vi "一体站流程自动启动.vi"(11 "参数":T1={"是否启用仪器"=FALSE, "CODMn"={"启动测量模式"={"测量模式"=enum."水样测量"}, "确定按钮"=TRUE}, "采水模式"=enum."使用采水泵"}) -> ()   [LabVIEW 2016, in "PLC.lvlib"]
uses:
  PLC.lvlib
panel:
  out "枚举":enum16{"初始化", "采配水启动", "等待", "配水", "排水", "结束"}(ring)
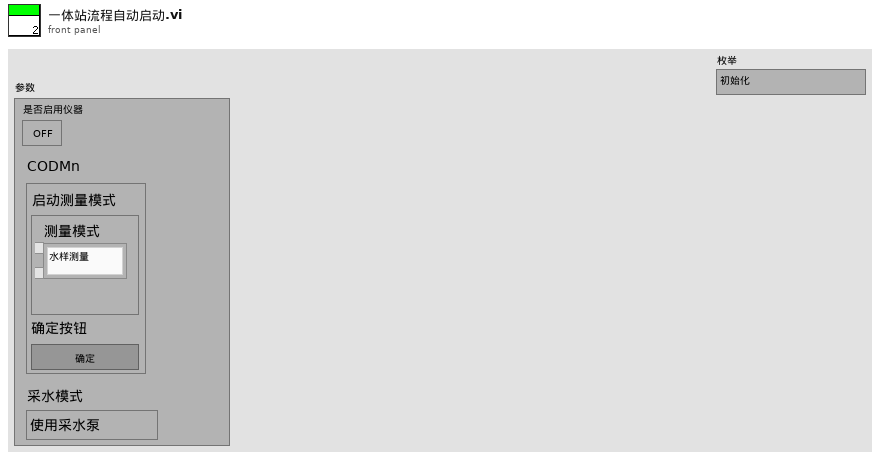
[diagram p1: front panel]
types:
  T1 = cluster{"是否启用仪器":bool, "CODMn":cluster{"启动测量模式":cluster{"测量模式":enum16{"水样测量", "标样核查", "零点核查", "加标回收", "平行样", "校零", "校标"}}, "确定按钮":bool}, "采水模式":enum16{"使用采水泵", "不使用采水泵"}}
  T2 = cluster{"命令":string, cluster{"starting address":u16, "holding register value":u16}}
  T3 = enum16{"待机", "启动氨氮", "氨氮测量中", "启动总磷", "总磷测量中", "结束"}
  T4 = cluster{"站号":u16, "量程切换":enum32{"H", "L", "AUTO"}, "控制命令":enum16{"启动测量", "标样核查", "零点核查", "跨度核查", "空白测试", "平行样测试", "加标回收", "空白校准", "标样校准", "初始化（清洗）", "停止测试", "仪器重启", "校时", "模式设置", "测量间隔设置", "盲样测试"}, "模式设置":enum16{"待机", "连续模式", "周期模式", "定点模式", "受控模式", "手动模式"}, "测量间隔":u16}
  T5 = cluster{"时间标识":timestamp, "设备":string, "日志信息":string}
  T6 = cluster{"测量模式":enum16{"待机", "水样测试", "标样核查", "零点核查", "跨度核查", "空白测试", "平行样测试", "加标回收", "空白校准", "标样校准", "初始化（清洗）"}, "数据标记表":string, "测量时间":dbl}
  T7 = enum16{"待机", "水样测试", "标样核查", "零点核查", "跨度核查", "空白测试", "平行样测试", "加标回收", "空白校准", "标样校准", "初始化（清洗）"}
  T8 = cluster{"R0":i16, "R1":i16, "R2":i16, "R3":i16, "R4":i16, "R5":i16, "R6":i16, "R7":i16, "R8":i16, "R9":i16, "R10":i16, "R11":i16, "R12":i16, "R13":i16, "R14":i16, "R15":i16, "R16":i16, "R17":i16, "R18":i16, "R19":i16, "R20":i16, "R21":i16, "R22":i16}
  T9 = enum32{"Bad", "Idle", "Run top level", "Running"}
  T10 = cluster{"测量模式":enum16{"水样测量", "标样核查", "零点核查", "加标回收", "平行样", "校零", "校标"}}
  T11 = cluster{"系统时间":timestamp, "工作状态":enum16{"空闲", "水样测试", "标样核查", "零点核查", "跨度核查", "空白测试", "平行样测试", "加标回收", "空白校准", "标样校准", "初始化（清洗）"}, "测量模式":enum16{"待机", "连续模式", "周期模式", "定点模式", "受控模式", "手动模式"}, "告警代码":enum16{"无告警", "缺试剂告警", "缺水样告警", "缺蒸馏水告警", "缺标液告警", "仪表漏液告警", "标定异常告警", "超量程告警", "加热异常", "低试剂预警", "超上限告警", "超下限告警", "仪表内部其他异常", "滴定异常告警", "电极异常告警", "量程切换告警", "参数设置告警", "PH电极电位异常", "电导率电极异常", "浊度光度异常", "溶解氧电极异常", "溶解氧光强异常", "温度异常告警", "PH异常告警", "溶解氧异常告警", "电导率异常告警", "浊度异常告警", "叶绿素异常告警", "藻密度异常告警", "蓝绿藻异常告警", "ORP异常告警", "氨氮异常告警", "清洁刷异常告警", "SD卡异常告警", "蓝牙异常告警", "Wifi异常告警", "流程异常告警"}, "故障代码":enum16{"无故障", "电机故障", "温度故障", "通讯故障", "滴定故障"}, "日志代码":u16, "软件版本":u16, "F0":sgl, "F1":sgl, "F2":sgl, "F3":sgl, "T":sgl, "H":sgl, "id":u16, "flowid":u16, "量程":u16}
  T12 = enum16{"空闲", "水样测试", "标样核查", "零点核查", "跨度核查", "空白测试", "平行样测试", "加标回收", "空白校准", "标样校准", "初始化（清洗）"}
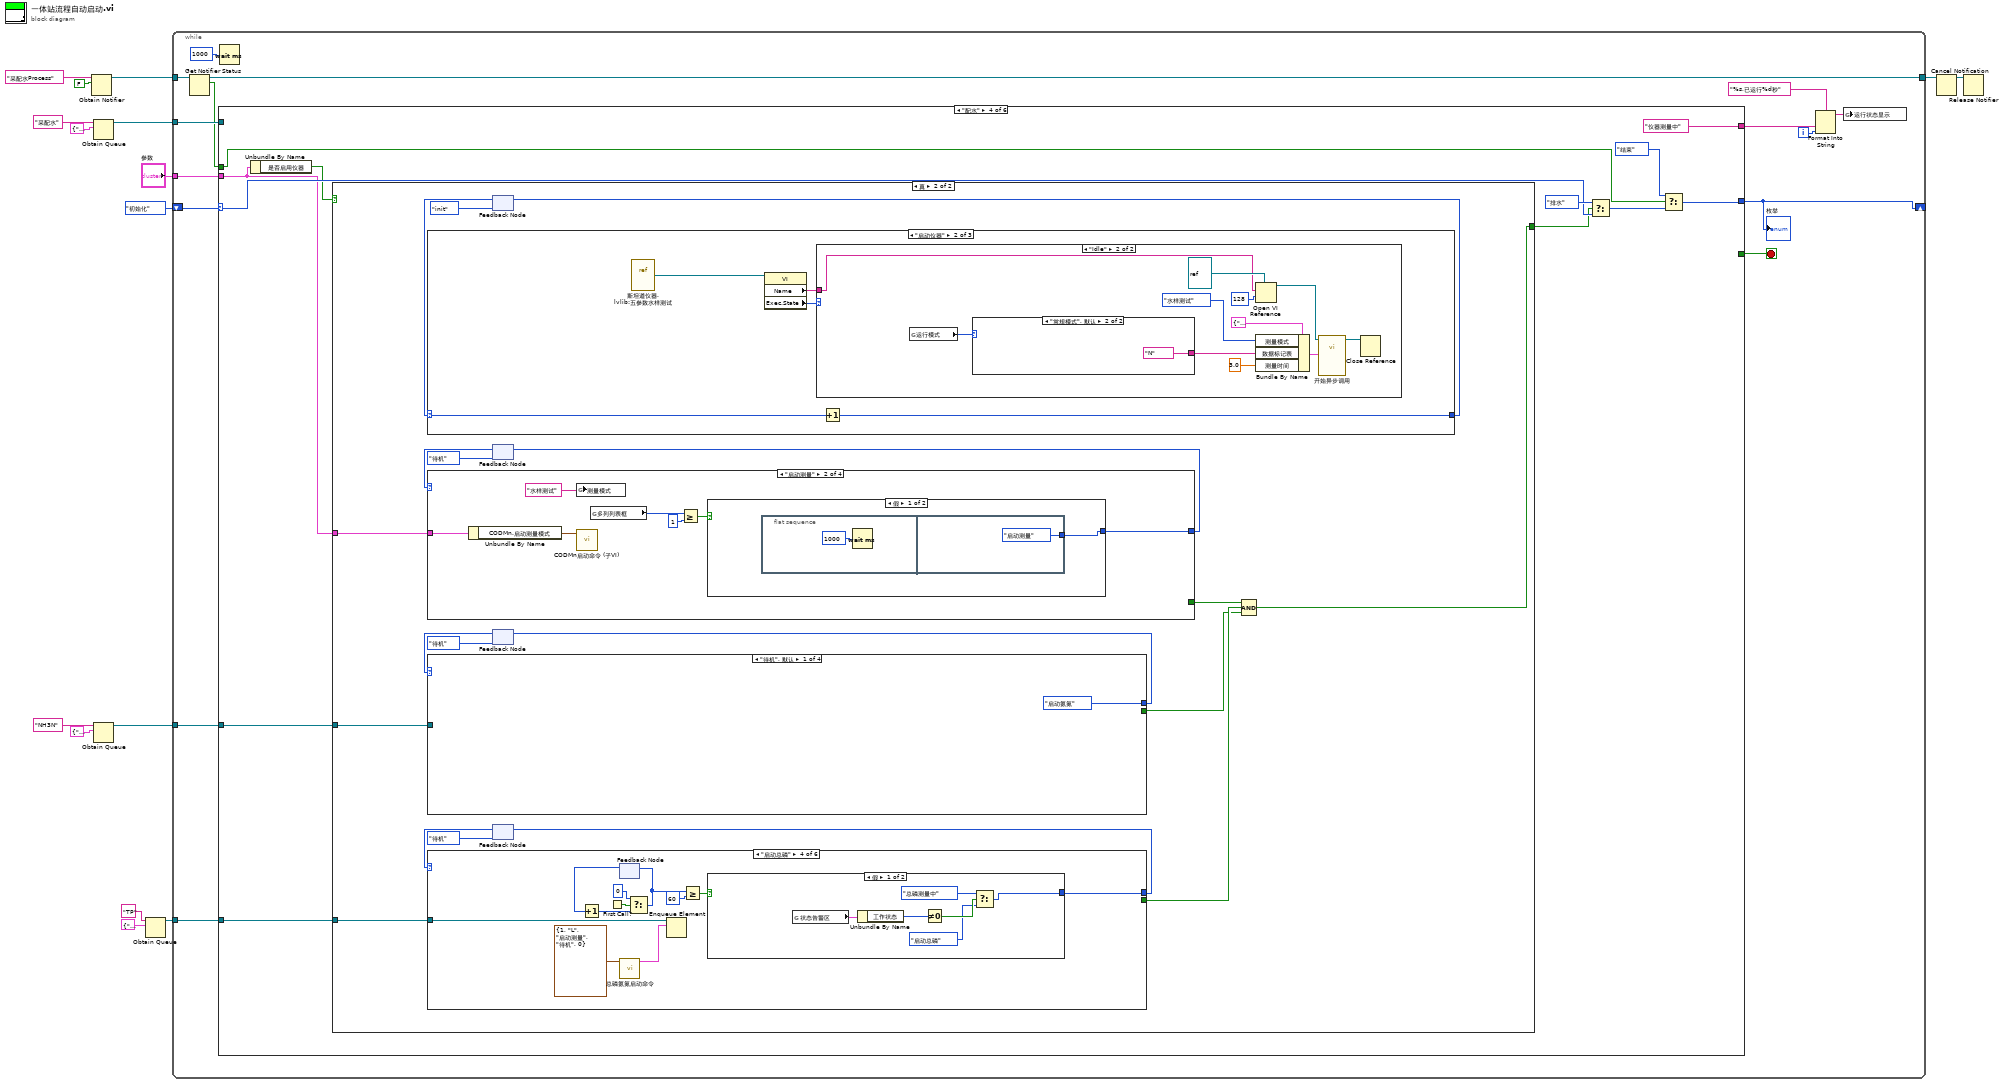
[diagram p0: block diagram]
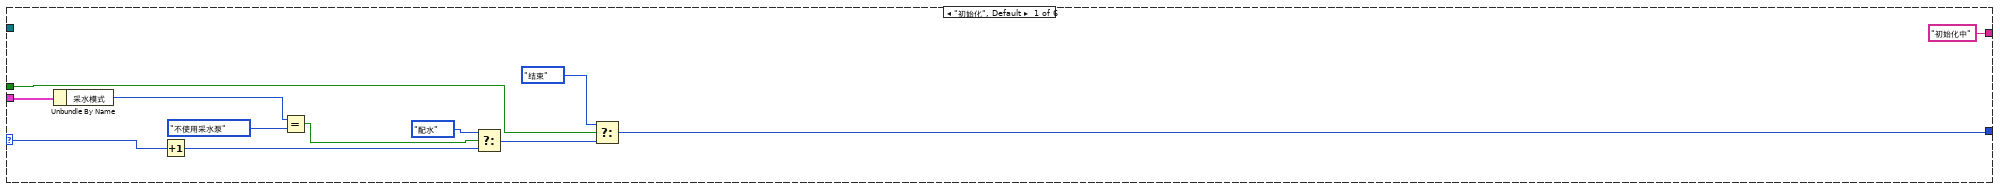
[diagram p2: hidden frame]
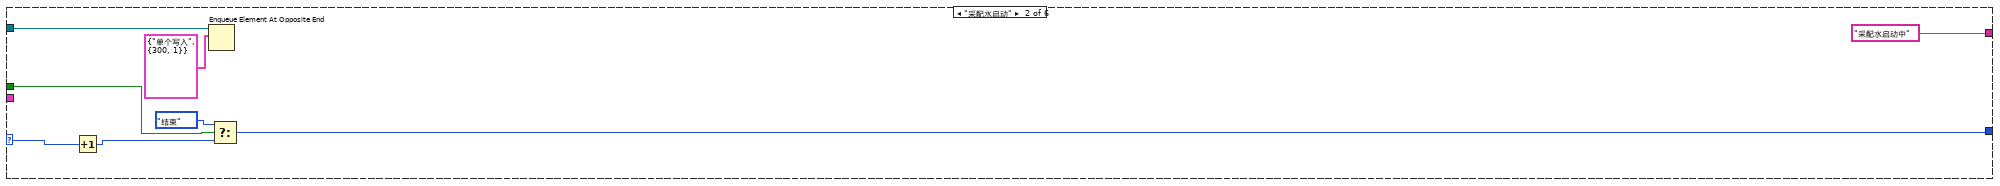
[diagram p3: hidden frame]
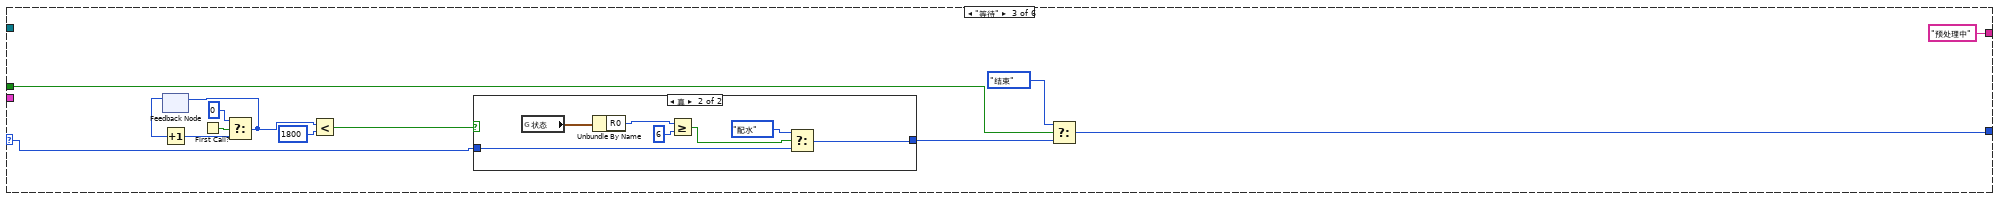
[diagram p4: hidden frame]
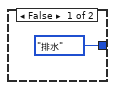
[diagram p5: hidden frame]
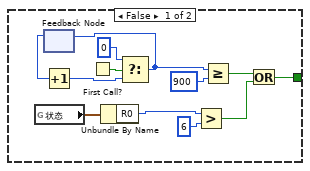
[diagram p6: hidden frame]
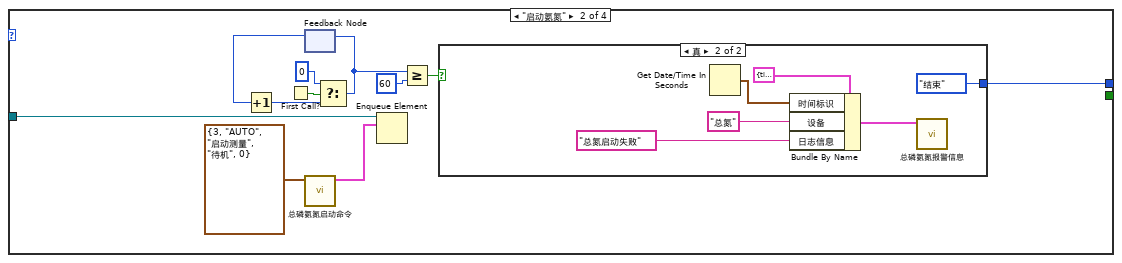
[diagram p7: hidden frame]
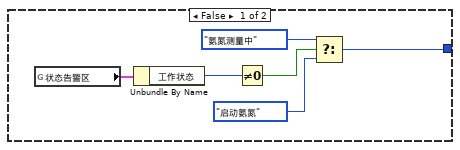
[diagram p8: hidden frame]
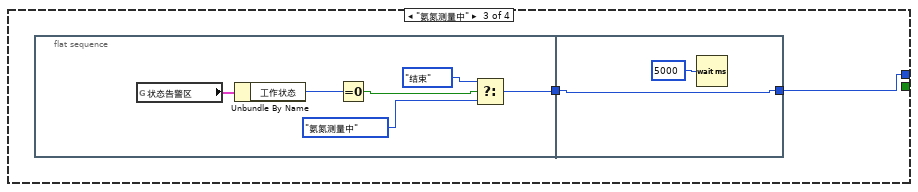
[diagram p9: hidden frame]
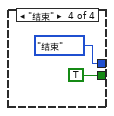
[diagram p10: hidden frame]
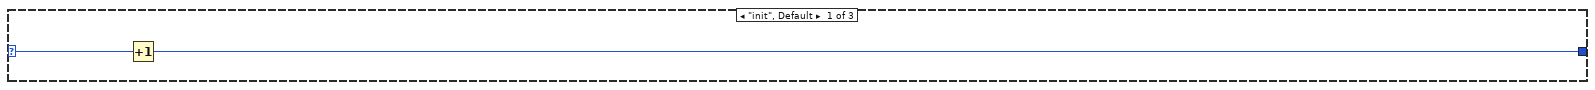
[diagram p11: hidden frame]
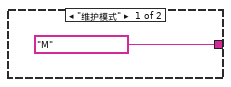
[diagram p13: hidden frame]
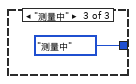
[diagram p14: hidden frame]
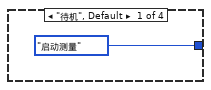
[diagram p15: hidden frame]
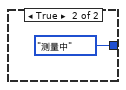
[diagram p16: hidden frame]
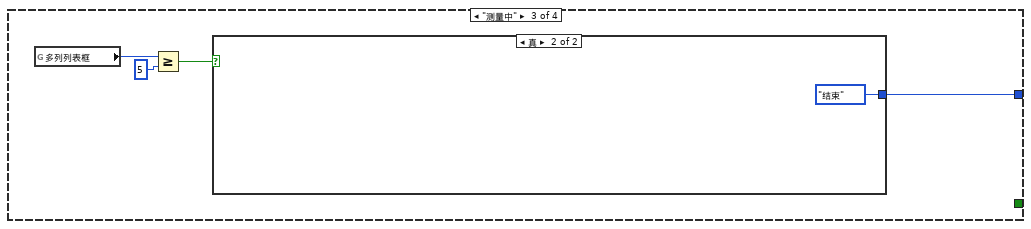
[diagram p17: hidden frame]
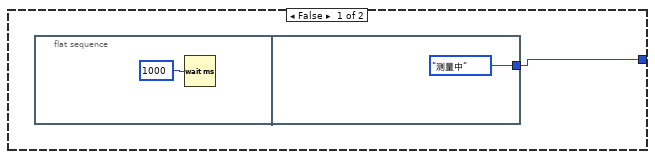
[diagram p18: hidden frame]
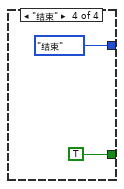
[diagram p19: hidden frame]
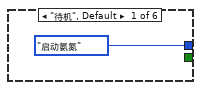
[diagram p20: hidden frame]
diagram:
  n1 = Obtain Notifier(name (unnamed)="采配水Process" ("名称（未命名）"), notification data type=FALSE) -> (notifier out=w6:refnum<notifier>)  [unwired: 2 in, 2 out]
  n2 = Obtain Queue(name (unnamed)="采配水" ("名称（未命名）"), element data type=cluster{"命令":string, "数据":variant} {"命令"="", "数据"=variant}) -> (queue out=w14:refnum<queue>)  [unwired: 3 in, 2 out]
  n3 = Obtain Queue(name (unnamed)="NH3N" ("名称（未命名）"), element data type=cluster{"命令":string, "data":variant} {"命令"="", "data"=variant}) -> (queue out=w1:refnum<queue>)  [unwired: 3 in, 2 out]
  n4 = Obtain Queue(name (unnamed)="TP" ("名称（未命名）"), element data type=cluster{"命令":string, "data":variant} {"命令"="", "data"=variant}) -> (queue out=w10:refnum<queue>)  [unwired: 3 in, 2 out]
  n5 = while {
    tunnel: w14 -> [w31]
    shift-right: [w29] -> _
    shift-left: enum16{"初始化", "采配水启动", "等待", "配水", "排水", "结束"}."初始化" ("枚举") -> [w30]
    tunnel: w10 -> [w27]
    tunnel: "参数" -> [w26]
    tunnel: w6 -> [w25]
    tunnel: [w24] -> w5
    tunnel: w1 -> [w23]
    i -> [w19]
    stop <- w22 stop-if-true
    n6 = Get Notifier Status(notifier=w25) -> (notifier out=w24:refnum<notifier>, current notification=w21:bool)  [unwired: 1 in, 3 out]
    n7 = case shown="\"配水\"" w30 {
      selector: w30 -> [w43 w49 w62 w83 w269 w278]
      tunnel: w31 -> [_ w50 _ _ w270 _]
      tunnel: [w33 w45 w52 w74 w264 w272] -> w29
      tunnel: [_ _ _ _ _ TRUE] -> w22
      tunnel: w27 -> [_ _ _ w82 _ _]
      tunnel: w26 -> [w42 _ _ w79 _ _]
      tunnel: w23 -> [_ _ _ w78 _ _]
      tunnel: w21 -> [w35 w47 w53 w73 w266 w274]
      tunnel: ["初始化中" ("输入 1") "采配水启动中" ("输入 1") "预处理中" ("输入 1") "仪器测量中" ("输入 1") "排水中" ("输入 1") "运行结束" ("输入 1")] -> w18
      frame "初始化", Default {
        n8 = Unbundle By Name(w42) -> ("采水模式"=w41:enum16{"使用采水泵", "不使用采水泵"})
        n9 = Increment(x=w43) -> (x+1=w37:enum16{"初始化", "采配水启动", "等待", "配水", "排水", "结束"})
        n10 = Equal?(x=w41, y=enum16{"使用采水泵", "不使用采水泵"}."不使用采水泵") -> (x = y?=w39:bool)
        n11 = Select(t=enum16{"初始化", "采配水启动", "等待", "配水", "排水", "结束"}."配水" ("枚举"), s=w39, f=w37) -> (s? t:f=w34:enum16{"初始化", "采配水启动", "等待", "配水", "排水", "结束"})
        n12 = Select(t=enum16{"初始化", "采配水启动", "等待", "配水", "排水", "结束"}."结束", s=w35, f=w34) -> (s? t:f=w33:enum16{"初始化", "采配水启动", "等待", "配水", "排水", "结束"})
      }
      frame "采配水启动" {
        n13 = Increment(x=w49) -> (x+1=w46:enum16{"初始化", "采配水启动", "等待", "配水", "排水", "结束"})
        n14 = Enqueue Element At Opposite End(queue=w50, element=T2 {"命令"="单个写入", {"starting address"=300, "holding register value"=1}} ("元素")) -> ()  [unwired: 2 in, 3 out]
        n15 = Select(t=enum16{"初始化", "采配水启动", "等待", "配水", "排水", "结束"}."结束", s=w47, f=w46) -> (s? t:f=w45:enum16{"初始化", "采配水启动", "等待", "配水", "排水", "结束"})
      }
      frame "等待" {
        n16 = feedback #1() -> (w59:i32)  [unwired: 1 in]
        n17 = Increment(x=w59) -> (x+1=w58:i32)
        n18 = First Call?() -> (First Call?: T/F=w60:bool)
        n19 = Select(t=0, s=w60, f=w58) -> (s? t:f=w57:i32)
        n20 = feedback-in #1(w57) -> ()
        n21 = Less?(x=w57, y=1800) -> (x < y?=w63:bool)
        n22 = case shown="真" w63 {
          tunnel: w62 -> [_ w67]
          tunnel: [enum16{"初始化", "采配水启动", "等待", "配水", "排水", "结束"}."排水" ("枚举") w66] -> w54
          frame False {
          }
          frame True {
            n23 = global read "采配水全局变量.vi" "状态"() -> (w72:T8)
            n24 = Unbundle By Name(w72) -> ("R0"=w71:i16)
            n25 = Greater Or Equal?(x=w71, y=i16 6) -> (x >= y?=w69:bool)
            n26 = Select(t=enum16{"初始化", "采配水启动", "等待", "配水", "排水", "结束"}."配水" ("枚举"), s=w69, f=w67) -> (s? t:f=w66:enum16{"初始化", "采配水启动", "等待", "配水", "排水", "结束"})
          }
        }
        n27 = Select(t=enum16{"初始化", "采配水启动", "等待", "配水", "排水", "结束"}."结束", s=w53, f=w54) -> (s? t:f=w52:enum16{"初始化", "采配水启动", "等待", "配水", "排水", "结束"})
      }
      frame "配水" {
        n28 = Unbundle By Name(w79) -> ("是否启用仪器"=w81:bool)
        n29 = case shown="真" w81 {
          tunnel: w82 -> [_ w112]
          tunnel: [w85 w97] -> w80
          tunnel: w79 -> [_ w108]
          tunnel: w78 -> [_ w101]
          frame False {
            n30 = global read "采配水全局变量.vi" "状态"() -> (w90:T8)
            n31 = feedback #2() -> (w94:i32)  [unwired: 1 in]
            n32 = Increment(x=w94) -> (x+1=w93:i32)
            n33 = First Call?() -> (First Call?: T/F=w95:bool)
            n34 = Unbundle By Name(w90) -> ("R0"=w89:i16)
            n35 = Select(t=0, s=w95, f=w93) -> (s? t:f=w91:i32)
            n36 = feedback-in #2(w91) -> ()
            n37 = Greater?(x=w89, y=i16 6) -> (0:w87:bool)
            n38 = Greater Or Equal?(x=w91, y=900) -> (x >= y?=w86:bool)
            n39 = Or(x=w86, y=w87) -> (x .or. y?=w85:bool)
          }
          frame True {
            n40 = feedback #3(enum16{"init", "启动仪器", "测量中"}."init") -> (w106:enum16{"init", "启动仪器", "测量中"})
            n41 = case shown="\"启动仪器\"" w106 {
              selector: w106 -> [w153 w158 _]
              tunnel: [w152 w157 enum16{"init", "启动仪器", "测量中"}."测量中"] -> w107
              frame "init", Default {
                n42 = Increment(x=w153) -> (x+1=w152:enum16{"init", "启动仪器", "测量中"})
              }
              frame "启动仪器" {
                n43 = vi-ref "斯坦道仪器.lvlib:五参数水样测试.vi"() -> (w155:refnum<vi>)
                n44 = property class="VI"(reference=w155) -> ("Name"=w154:string, "Exec.State"=w156:T9)  [unwired: 1 in, 2 out]
                n45 = case shown="\"Idle\"" w156 {
                  tunnel: w154 -> [_ w165]
                  frame "Bad", Default {
                  }
                  frame "Idle" {
                    n46 = global read "系统变量.vi" "运行模式"() -> (w160:enum16{"维护模式", "常规模式", "应急模式", "质控模式"})
                    n47 = case shown="\"常规模式\", 默认" w160 {
                      tunnel: ["M" ("数据标记表") "N" ("数据标记表")] -> w159
                      frame "维护模式" {
                      }
                      frame "常规模式", Default {
                      }
                    }
                    n48 = Bundle By Name(cluster=T6 {"测量模式"=enum."待机", "数据标记表"="", "测量时间"=0.0} ("启动参数"), "测量模式"=T7."水样测试", "数据标记表"=w159, "测量时间"=3.0) -> (w161:T6)
                    n49 = Open VI Reference(type specifier VI Refnum (for type only)=refnum<vi> refnum ("类型说明符VI引用句柄（仅用于类型）"), vi path=w165, options=128 ("选项")) -> (vi reference=w164:refnum<vi>)  [unwired: 3 in, 1 out]
                    n50 = call-by-ref "开始异步调用"(reference=w164, "启动参数"=w161) -> (reference out=w163:refnum<vi>)  [unwired: 12 in, 1 out]
                    n51 = Close Reference(reference=w163) -> ()  [unwired: 1 in, 1 out]
                  }
                }
                n52 = Increment(x=w158) -> (x+1=w157:enum16{"init", "启动仪器", "测量中"})
              }
              frame "测量中" {
              }
            }
            n53 = feedback-in #3(w107) -> ()
            n54 = feedback #4(enum16{"待机", "启动测量", "测量中", "结束"}."待机") -> (w110:enum16{"待机", "启动测量", "测量中", "结束"})
            n55 = case shown="\"启动测量\"" w110 {
              tunnel: [enum16{"待机", "启动测量", "测量中", "结束"}."启动测量" w177 w186 enum16{"待机", "启动测量", "测量中", "结束"}."结束"] -> w109
              tunnel: w108 -> [_ w180 _ _]
              tunnel: [_ _ _ TRUE] -> w100
              frame "待机", Default {
              }
              frame "启动测量" {
                n56 = Unbundle By Name(w180) -> ("CODMn.启动测量模式"=w175:T10)
                n57 = global write "COD测量模式全局.vi" "测量模式"("水样测试" ("测量模式")) -> ()
                n58 = call "CODMn启动命令 (子VI).vi"("启动测量模式"=w175) -> ()  [unwired: 11 in]
                n59 = global read "运行时序全局变量.vi" "多列列表框"() -> (w176:i32)
                n60 = Greater Or Equal?(x=w176, y=1) -> (x >= y?=w178:bool)
                n61 = case shown="假" w178 {
                  tunnel: [w181 enum16{"待机", "启动测量", "测量中", "结束"}."测量中"] -> w177
                  frame False {
                    n62 = flat-sequence {
                      tunnel: [enum16{"待机", "启动测量", "测量中", "结束"}."启动测量"] -> w181
                      frame #0 {
                        n63 = Wait (ms)(milliseconds to wait=u32 1000 ("等待时间（毫秒）")) -> ()  [unwired: 1 out]
                      }
                      frame #1 {
                      }
                    }
                  }
                  frame True {
                  }
                }
              }
              frame "测量中" {
                n64 = global read "运行时序全局变量.vi" "多列列表框"() -> (w185:i32)
                n65 = Greater Or Equal?(x=w185, y=5) -> (x >= y?=w187:bool)
                n66 = case shown="真" w187 {
                  tunnel: [w189 enum16{"待机", "启动测量", "测量中", "结束"}."结束"] -> w186
                  frame False {
                    n67 = flat-sequence {
                      tunnel: [enum16{"待机", "启动测量", "测量中", "结束"}."测量中"] -> w189
                      frame #0 {
                        n68 = Wait (ms)(milliseconds to wait=u32 1000 ("等待时间（毫秒）")) -> ()  [unwired: 1 out]
                      }
                      frame #1 {
                      }
                    }
                  }
                  frame True {
                  }
                }
              }
              frame "结束" {
              }
            }
            n69 = feedback-in #4(w109) -> ()
            n70 = feedback #5(T3."待机") -> (w103:T3)
            n71 = case shown="\"待机\", 默认" w103 {
              tunnel: [T3."启动氨氮" w126 w141 T3."结束"] -> w104
              tunnel: w101 -> [_ w127 _ _]
              tunnel: [_ _ _ TRUE] -> w98
              frame "待机", Default {
              }
              frame "启动氨氮" {
                n72 = First Call?() -> (First Call?: T/F=w124:bool)
                n73 = feedback #6() -> (w123:i32)  [unwired: 1 in]
                n74 = Increment(x=w123) -> (x+1=w122:i32)
                n75 = call "总磷氨氮启动命令.vi"("参数"=T4 {"站号"=3, "量程切换"=enum."AUTO", "控制命令"=enum."启动测量", "模式设置"=enum."待机", "测量间隔"=0}) -> ("启动命令"=w118:cluster{"命令":string, "data":variant})  [unwired: 10 in]
                n76 = Select(t=0, s=w124, f=w122) -> (s? t:f=w121:i32)
                n77 = feedback-in #6(w121) -> ()
                n78 = Enqueue Element(queue=w127, element=w118) -> ()  [unwired: 2 in, 3 out]
                n79 = Greater Or Equal?(x=w121, y=60) -> (x >= y?=w119:bool)
                n80 = case shown="真" w119 {
                  tunnel: [w130 T3."结束"] -> w126
                  frame False {
                    n81 = global read "VAR总磷氨氮全局变量.vi" "状态告警区"() -> (w133:T11)
                    n82 = Unbundle By Name(w133) -> ("工作状态"=w132:T12)
                    n83 = Not Equal To 0?(x=w132) -> (x != 0?=w131:bool)
                    n84 = Select(t=T3."氨氮测量中", s=w131, f=T3."启动氨氮") -> (s? t:f=w130:T3)
                  }
                  frame True {
                    n85 = Get Date/Time In Seconds() -> (seconds since 1Jan1904=w138:timestamp)
                    n86 = Bundle By Name(cluster=T5 {"时间标识"=timestamp(0 s since 1904-01-01), "设备"="", "日志信息"=""} ("data in"), "时间标识"=w138, "设备"="总氮", "日志信息"="总氮启动失败") -> (w134:T5)
                    n87 = call "总磷氨氮报警信息.vi"("data in"=w134) -> ()  [unwired: 11 in]
                  }
                }
              }
              frame "氨氮测量中" {
                n88 = flat-sequence {
                  tunnel: [w145] -> w140
                  tunnel: [w149] -> w141
                  tunnel: w140 -> [w149]
                  frame #0 {
                    n89 = global read "VAR总磷氨氮全局变量.vi" "状态告警区"() -> (w146:T11)
                    n90 = Unbundle By Name(w146) -> ("工作状态"=w147:T12)
                    n91 = Equal To 0?(x=w147) -> (x = 0?=w144:bool)
                    n92 = Select(t=T3."结束", s=w144, f=T3."氨氮测量中") -> (s? t:f=w145:T3)
                  }
                  frame #1 {
                    n93 = Wait (ms)(milliseconds to wait=u32 5000 ("等待时间（毫秒）")) -> ()  [unwired: 1 out]
                  }
                }
              }
              frame "结束" {
              }
            }
            n94 = feedback-in #5(w104) -> ()
            n95 = feedback #7(T3."待机") -> (w114:T3)
            n96 = case shown="\"启动总磷\"" w114 {
              tunnel: [T3."启动氨氮" w205 w219 w238 w252 T3."结束"] -> w113
              tunnel: w112 -> [_ w206 _ w239 _ _]
              tunnel: [_ _ _ _ _ TRUE] -> w99
              frame "待机", Default {
              }
              frame "启动氨氮" {
                n97 = First Call?() -> (First Call?: T/F=w203:bool)
                n98 = feedback #8() -> (w202:i32)  [unwired: 1 in]
                n99 = Increment(x=w202) -> (x+1=w201:i32)
                n100 = call "总磷氨氮启动命令.vi"("参数"=T4 {"站号"=2, "量程切换"=enum."L", "控制命令"=enum."启动测量", "模式设置"=enum."待机", "测量间隔"=0}) -> ("启动命令"=w197:cluster{"命令":string, "data":variant})  [unwired: 10 in]
                n101 = Select(t=0, s=w203, f=w201) -> (s? t:f=w200:i32)
                n102 = feedback-in #8(w200) -> ()
                n103 = Enqueue Element(queue=w206, element=w197) -> ()  [unwired: 2 in, 3 out]
                n104 = Greater Or Equal?(x=w200, y=60) -> (x >= y?=w198:bool)
                n105 = case shown="假" w198 {
                  tunnel: [w209 T3."启动总磷"] -> w205
                  frame False {
                    n106 = global read "VAR总磷氨氮全局变量.vi" "状态告警区"() -> (w212:T11)
                    n107 = Unbundle By Name(w212) -> ("工作状态"=w211:T12)
                    n108 = Not Equal To 0?(x=w211) -> (x != 0?=w210:bool)
                    n109 = Select(t=T3."氨氮测量中", s=w210, f=T3."启动氨氮") -> (s? t:f=w209:T3)
                  }
                  frame True {
                    n110 = Get Date/Time In Seconds() -> (seconds since 1Jan1904=w217:timestamp)
                    n111 = Bundle By Name(cluster=T5 {"时间标识"=timestamp(0 s since 1904-01-01), "设备"="", "日志信息"=""} ("data in"), "时间标识"=w217, "设备"="总氮", "日志信息"="总氮启动失败") -> (w213:T5)
                    n112 = call "总磷氨氮报警信息.vi"("data in"=w213) -> ()  [unwired: 11 in]
                  }
                }
              }
              frame "氨氮测量中" {
                n113 = global read "VAR总磷氨氮全局变量.vi" "状态告警区"() -> (w222:T11)
                n114 = Unbundle By Name(w222) -> ("工作状态"=w221:T12, "id"=w220:u16)
                n115 = case shown="默认" w221 {
                  tunnel: w220 -> [_ w226]
                  tunnel: [T3."启动总磷" w225] -> w219
                  frame "空闲" {
                    n116 = Wait (ms)(milliseconds to wait=u32 5000 ("等待时间（毫秒）")) -> ()  [unwired: 1 out]
                  }
                  frame Default {
                    n117 = case shown="131" w226 {
                      tunnel: [T3."氨氮测量中" T3."总磷测量中"] -> w225
                      frame 76, Default {
                      }
                      frame 131 {
                      }
                    }
                  }
                }
              }
              frame "启动总磷" {
                n118 = First Call?() -> (First Call?: T/F=w236:bool)
                n119 = feedback #9() -> (w235:i32)  [unwired: 1 in]
                n120 = Increment(x=w235) -> (x+1=w234:i32)
                n121 = call "总磷氨氮启动命令.vi"("参数"=T4 {"站号"=1, "量程切换"=enum."L", "控制命令"=enum."启动测量", "模式设置"=enum."待机", "测量间隔"=0}) -> ("启动命令"=w230:cluster{"命令":string, "data":variant})  [unwired: 10 in]
                n122 = Select(t=0, s=w236, f=w234) -> (s? t:f=w233:i32)
                n123 = feedback-in #9(w233) -> ()
                n124 = Enqueue Element(queue=w239, element=w230) -> ()  [unwired: 2 in, 3 out]
                n125 = Greater Or Equal?(x=w233, y=60) -> (x >= y?=w231:bool)
                n126 = case shown="假" w231 {
                  tunnel: [w242 T3."结束"] -> w238
                  frame False {
                    n127 = global read "VAR总磷氨氮全局变量.vi" "状态告警区"() -> (w243:T11)
                    n128 = Unbundle By Name(w243) -> ("工作状态"=w244:T12)
                    n129 = Not Equal To 0?(x=w244) -> (x != 0?=w245:bool)
                    n130 = Select(t=T3."总磷测量中", s=w245, f=T3."启动总磷") -> (s? t:f=w242:T3)
                  }
                  frame True {
                    n131 = Get Date/Time In Seconds() -> (seconds since 1Jan1904=w251:timestamp)
                    n132 = Bundle By Name(cluster=T5 {"时间标识"=timestamp(0 s since 1904-01-01), "设备"="", "日志信息"=""} ("data in"), "时间标识"=w251, "设备"="总磷", "日志信息"="总磷启动失败") -> (w246:T5)
                    n133 = call "总磷氨氮报警信息.vi"("data in"=w246) -> ()  [unwired: 11 in]
                  }
                }
              }
              frame "总磷测量中" {
                n134 = global read "VAR总磷氨氮全局变量.vi" "状态告警区"() -> (w255:T11)
                n135 = Unbundle By Name(w255) -> ("工作状态"=w254:T12, "id"=w253:u16)
                n136 = case shown="默认" w254 {
                  tunnel: w253 -> [_ w259]
                  tunnel: [T3."结束" w258] -> w252
                  frame "空闲" {
                    n137 = Wait (ms)(milliseconds to wait=u32 5000 ("等待时间（毫秒）")) -> ()  [unwired: 1 out]
                  }
                  frame Default {
                    n138 = case shown="131" w259 {
                      tunnel: [T3."氨氮测量中" T3."总磷测量中"] -> w258
                      frame 76, Default {
                      }
                      frame 131 {
                      }
                    }
                  }
                }
              }
              frame "结束" {
              }
            }
            n139 = feedback-in #7(w113) -> ()
            n140 = Compound Arithmetic op=AND ("复合运算")(w100, w99, w98) -> (w97:bool)
          }
        }
        n141 = Select(t=enum16{"初始化", "采配水启动", "等待", "配水", "排水", "结束"}."排水" ("枚举"), s=w80, f=w83) -> (s? t:f=w75:enum16{"初始化", "采配水启动", "等待", "配水", "排水", "结束"})
        n142 = Select(t=enum16{"初始化", "采配水启动", "等待", "配水", "排水", "结束"}."结束", s=w73, f=w75) -> (s? t:f=w74:enum16{"初始化", "采配水启动", "等待", "配水", "排水", "结束"})
      }
      frame "排水" {
        n143 = Increment(x=w269) -> (x+1=w265:enum16{"初始化", "采配水启动", "等待", "配水", "排水", "结束"})
        n144 = Enqueue Element At Opposite End(queue=w270, element=T2 {"命令"="单个写入", {"starting address"=303, "holding register value"=1}} ("元素")) -> ()  [unwired: 2 in, 3 out]
        n145 = Select(t=enum16{"初始化", "采配水启动", "等待", "配水", "排水", "结束"}."结束", s=w266, f=w265) -> (s? t:f=w264:enum16{"初始化", "采配水启动", "等待", "配水", "排水", "结束"})
      }
      frame "结束" {
        n146 = Increment(x=w278) -> (x+1=w273:enum16{"初始化", "采配水启动", "等待", "配水", "排水", "结束"})
        n147 = Select(t=enum16{"初始化", "采配水启动", "等待", "配水", "排水", "结束"}."结束", s=w274, f=w273) -> (s? t:f=w272:enum16{"初始化", "采配水启动", "等待", "配水", "排水", "结束"})
      }
    }
    "枚举" <- w29
    n148 = Wait (ms)(milliseconds to wait=u32 1000 ("等待时间（毫秒）")) -> ()  [unwired: 1 out]
    n149 = Format Into String(format string="%s,已运行%d秒" ("格式字符串"), w18, w19) -> (resulting string=w17:string)  [unwired: 2 in, 1 out]
    n150 = global write "采配水全局变量.vi" "运行状态显示"(w17) -> ()
  }
  n151 = Cancel Notification(0:w5) -> (8:w4:refnum<notifier>)  [unwired: 1 in, 2 out]
  n152 = Release Notifier(notifier=w4) -> ()  [unwired: 2 in, 3 out]
